vi "VI Inspector.vi"() -> ()   [LabVIEW 2016]
panel:
  in  "options":i32 format="%.0x"
  out "Metrics:Block Diagram Loaded":bool
  out "Modifications:Block Diagram Mods Bitset":u32
  out "Modifications:Front Panel Mods Bitset":u32
  out "Modifications:VI Modifications Bitset":u64 format="%x"
  out "Contains Compiled Code":bool
  out "Execution:State":T1(ring)
  in  "File Path Control":path
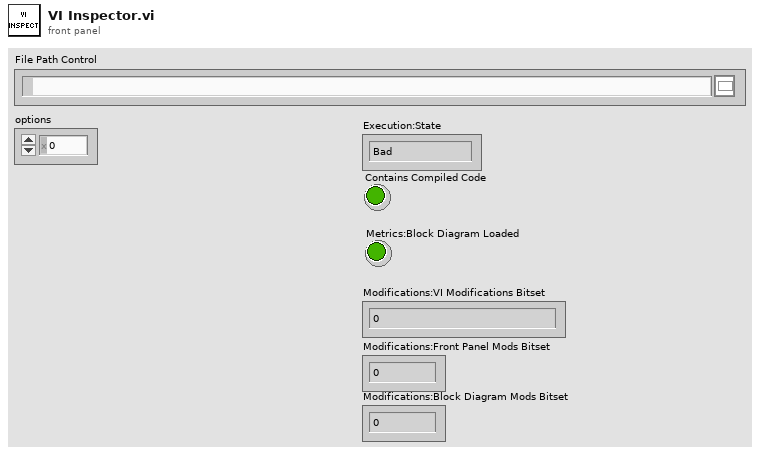
[diagram p1: front panel]
types:
  T1 = enum32{"Bad", "Idle", "Run top level", "Running"}
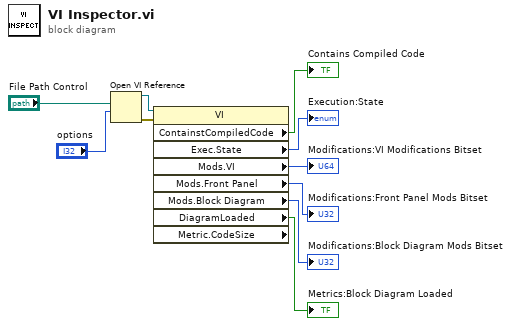
[diagram p0: block diagram]
diagram:
  n1 = Open VI Reference(vi path="File Path Control", options="options") -> (vi reference=w10:refnum<vi>, error out=w9:errorcluster)  [unwired: 4 in]
  n2 = property class="VI" props=["ContainstCompiledCode", "Exec.State", "Mods.VI", "Mods.Front Panel", "Mods.Block Diagram", "DiagramLoaded", "Metric.CodeSize"](reference=w10, error in=w9) -> ("ContainstCompiledCode"=→"Contains Compiled Code":bool, "Exec.State"=→"Execution:State":T1, "Mods.VI"=→"Modifications:VI Modifications Bitset":u64, "Mods.Front Panel"=→"Modifications:Front Panel Mods Bitset":u32, "Mods.Block Diagram"=→"Modifications:Block Diagram Mods Bitset":u32, "DiagramLoaded"=→"Metrics:Block Diagram Loaded":bool)  [unwired: 3 out]
